vi "Get User Events.vi"(8 "error in (no error)":errorcluster, 11 "Model in":refnum<class "Model.lvclass">) -> (0 "error out":errorcluster, 2 "User Events.lvclass":refnum<class "User Events.lvclass">, 3 "Model out":refnum<class "Model.lvclass">)   [LabVIEW 2016, in "Model.lvclass"]
uses:
  Model.lvclass
  User Events/User Events.lvclass
  Model.lvclass/Model.ctl
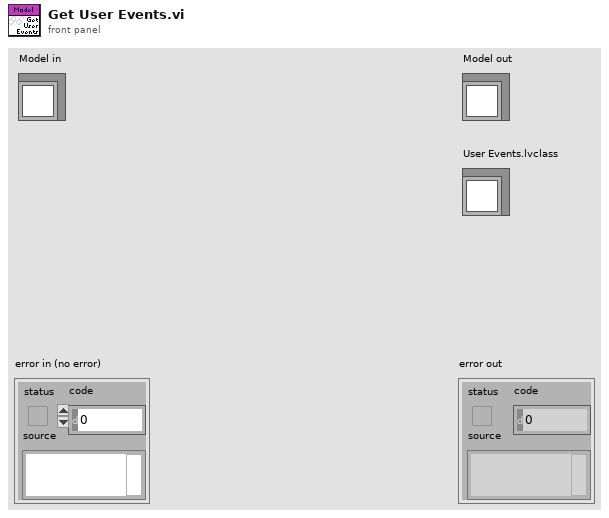
[diagram p1: front panel]
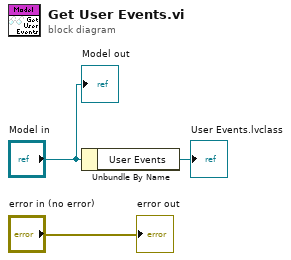
[diagram p0: block diagram]
diagram:
  n1 = Unbundle By Name("Model in") -> ("User Events"=→"User Events.lvclass":refnum<class "User Events.lvclass">)
  "error out" <- "error in (no error)"
  "Model out" <- "Model in"
